vi "Update Motor State Value.vi"(8 "error in (no error)":errorcluster, 9 "state mode":T1 items=["undefined", "angle", "velocity"], 10 "value":dbl, 11 "motorcommunication in":refnum<class "NI_Robotics_Motor Communication Ref.lvclass">) -> (0 "error out":errorcluster, 1 "failed?":bool, 3 "motor communication out":refnum<class "NI_Robotics_Motor Communication Ref.lvclass">)   [LabVIEW 2017, in "NI_Robotics_Motor Communication Ref.lvclass"]
uses:
  <vilib>/robotics/Actuation/Motor Communication Ref/NI_Robotics_Motor Communication Ref.lvclass
  <vilib>/robotics/Actuation/Motor Communication/Motor State Mode.ctl
  <vilib>/robotics/Actuation/Motor Communication Ref/NI_Robotics_Motor Communication Ref.lvclass/NI_Robotics_Motor Communication Ref.ctl
  <vilib>/robotics/Actuation/Motor Communication/Write to Motor State.vi
  <vilib>/robotics/Actuation/Motor Communication/NI_Robotics_Motor Communication.lvclass
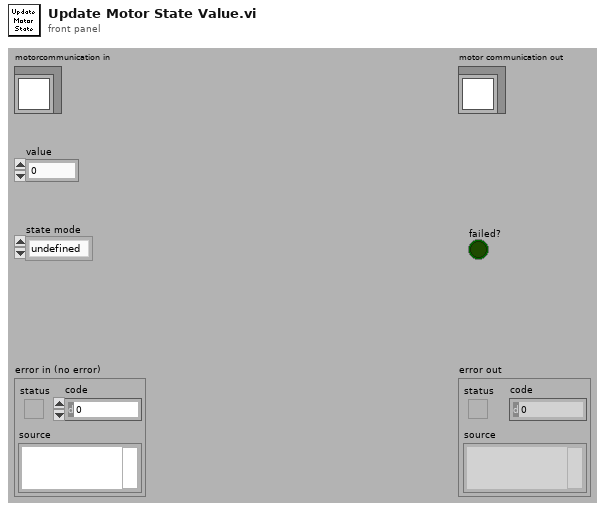
[diagram p1: front panel]
types:
  T1 = typedef "NI_Robotics_Motor Communication.lvclass/Motor State Mode.ctl" = u16
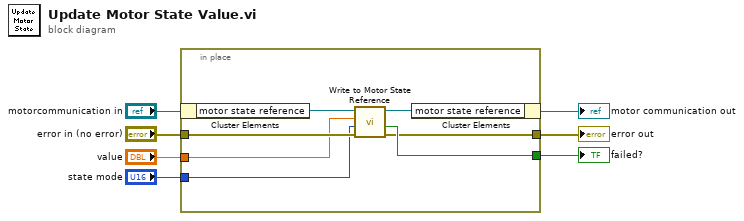
[diagram p0: block diagram]
diagram:
  n1 = in-place {
    in-place-border: [w12] -> w6
    in-place-border: "error in (no error)" -> [w11]
    in-place-border: "value" -> [w10]
    in-place-border: "state mode" -> [w9]
    in-place-border: [w8] -> w7
    n2 = in-place-cluster #1("motorcommunication in") -> ("motor state reference"=w14:refnum<data-value>)
    n3 = call <vilib>:"Write to Motor State Reference.vi"("error in (no error)"=w11, "state mode"=w9, "value"=w10, "motor state ref in"=w14) -> ("error out"=w8:errorcluster, "failed?"=w12:bool, "motor state ref out"=w13:refnum<data-value>)  [unwired: 5 in]
    n4 = in-place-cluster #1("motor state reference"=w13) -> (→"motor communication out":refnum<class "NI_Robotics_Motor Communication Ref.lvclass">)
  }
  "error out" <- w7
  "failed?" <- w6
